vi "ReadModule.vi"(11 "VISA Refnum in":refnum<visa-resource-name>) -> (0 "error out":errorcluster, 1 "unsigned byte array":u8[](array[numeric]), 2 "Boolean":bool, 3 "VISA Refnum out":refnum<visa-resource-name>)   [LabVIEW 2013]
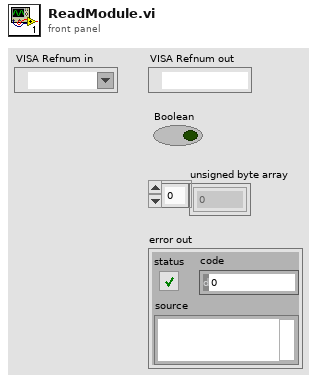
[diagram p1: front panel]
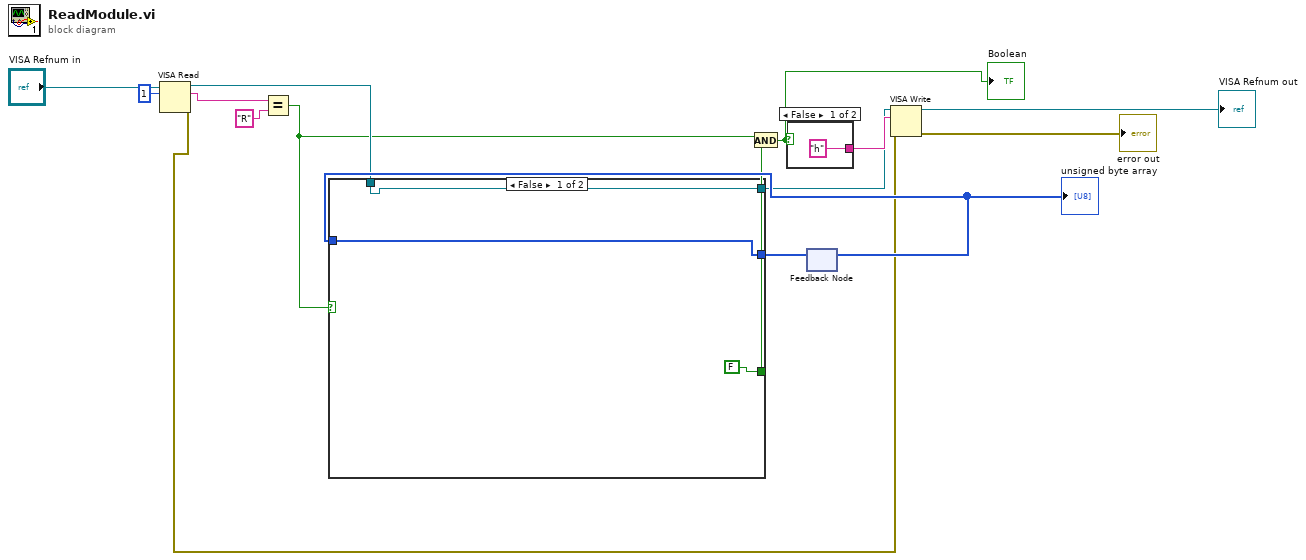
[diagram p0: block diagram]
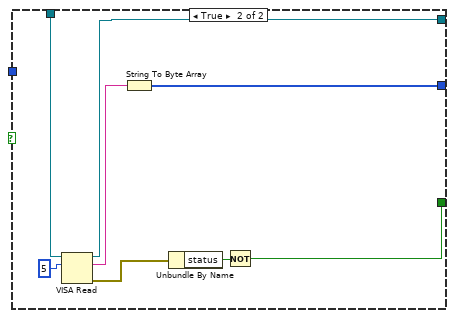
[diagram p2: hidden frame]
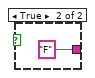
[diagram p3: hidden frame]
diagram:
  n1 = VISA Read(VISA resource name="VISA Refnum in", byte count=u32 1) -> (VISA resource name out=w5:refnum<visa-resource-name>, read buffer=w11:string, error out=w2:errorcluster)  [unwired: 1 in, 1 out]
  n2 = Equal?(x=w11, y="R") -> (x = y?=w1:bool)
  n3 = feedback #1() -> (w14:u8[])  [unwired: 1 in]
  "unsigned byte array" <- w14
  n4 = case shown="False" w1 {
    tunnel: w5 -> [w18 w24]
    tunnel: [w18 w22] -> w8
    tunnel: [FALSE w20] -> w10
    tunnel: [w16 w19] -> w13
    tunnel: w14 -> [w16 _]
    frame False {
    }
    frame True {
      n5 = VISA Read(VISA resource name=w24, byte count=u32 5) -> (VISA resource name out=w22:refnum<visa-resource-name>, read buffer=w25:string, error out=w23:errorcluster)  [unwired: 1 in, 1 out]
      n6 = String To Byte Array(string=w25) -> (unsigned byte array=w19:u8[])
      n7 = Unbundle By Name(w23) -> ("status"=w21:bool)
      n8 = Not(x=w21) -> (.not. x?=w20:bool)
    }
  }
  n9 = And(x=w1, y=w10) -> (x .and. y?=w15:bool)
  "Boolean" <- w15
  n10 = case shown="False" w15 {
    tunnel: ["h" ("write buffer") "F" ("write buffer")] -> w9
    frame False {
    }
    frame True {
    }
  }
  n11 = feedback-in #1(w13) -> ()
  n12 = VISA Write(VISA resource name=w8, write buffer=w9, error in (no error)=w2) -> (VISA resource name out=→"VISA Refnum out":refnum<visa-resource-name>, error out=→"error out":errorcluster)  [unwired: 1 out]
